vi "Visualise STL file and Octree.vi"() -> ()   [LabVIEW 2017]
doc: "Interactive tool to inspect an STL file and build the Octree for the STL file and check the resulting output. The Octree resolution may be interactively adjusted or set to automatic. The number of branch levels and nodes depends on the geometry, however a rough guide would be to aim for between 5 and 7 branch levels and order 10k nodes."
uses:
  <vilib>/Utility/miscctls.llb/LV3DPointTypeDef.ctl
  <vilib>/Utility/miscctls.llb/LVRGBAColorTypeDef.ctl
  Typedefs/TreeNodeBox.ctl
  Typedefs/Quad.ctl
  Typedefs/Quadplane enum.ctl
  Subroutines/Dot product.vi
panel:
  out "error out":errorcluster
  in  "Camera Controller:Type":T1(ring)=enum."Oriented"
  in  "Autocalc Octree resolution":bool=TRUE
  out "Branch levels":i32
  in  "Scale to unit sphere (render only)":bool
  in  "Octree file path":path=path "C:/EnFlo Software/Anemometry/Anemometry Sub Vis/Collision_Detection/Triangles/Example files/DIPLOS array.oct"
  in  "Render mode":u16(ring)=3 items=["Inherit Value", "Points", "Wireframe", "Polygons"]
  in  "Build Octree":bool
  in  "Draw populated leaf nodes only":bool=TRUE
  out "Number of triangles":u32
  in  "STL file path":path=path "C:/EnFlo Software/Anemometry/Anemometry Sub Vis/Collision_Detection/Triangles/Example files/DIPLOS array.stl"
  in  "Render window":bool=TRUE
  out "Number of Octree nodes":i32
  in  "Octree resolution (model units)":sgl=100.0
  out "Pmin (x, y, z)":sgl[](array[numeric])
  out "Pmax (x, y, z)":sgl[](array[numeric])
  in  "Up Direction":T2={"X"=0.0, "Y"=0.0, "Z"=1.0}
  in  "Target":T2
  in  "Camera Position":T2={"X"=3000.0, "Y"=0.0, "Z"=1000.0}
  out "3D Picture":refnum<vi>(3d-picture)
  # "To view model alone, uncheck \"Build Octree\" and empty \"Octree binary path\".\nTo load Octree after build, uncheck \"Build Octree\"."
  # "PN 03/02/2015"
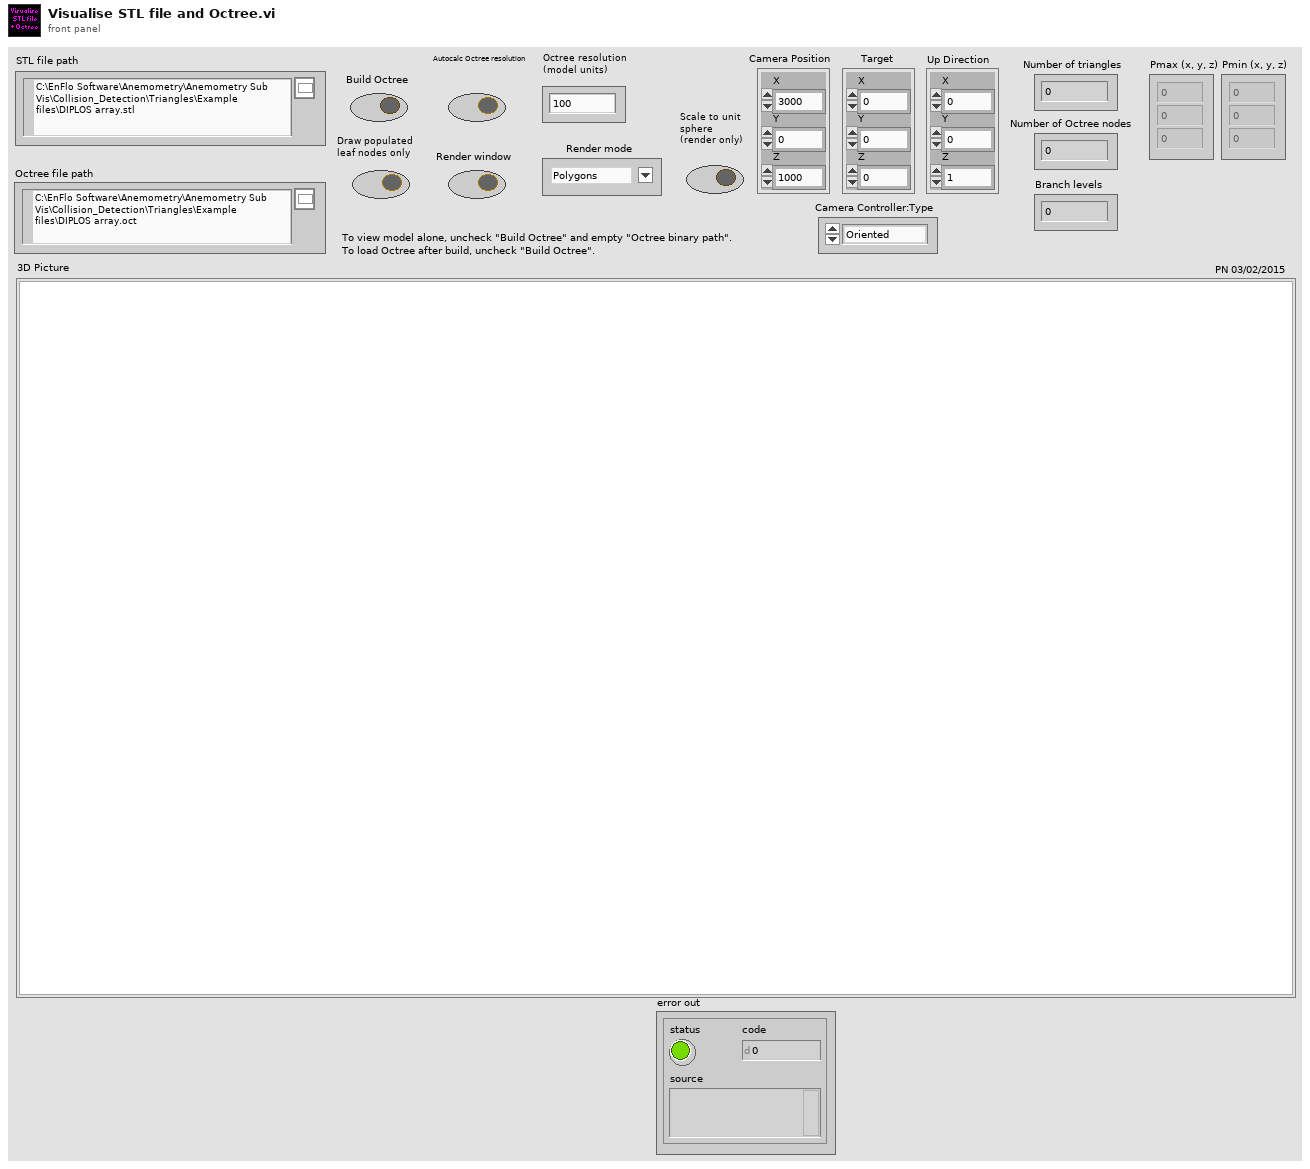
[diagram p1: front panel]
types:
  T1 = enum16{"None", "Spherical", "Flying", "Oriented"}
  T2 = typedef "LV3DPointTypeDef.ctl" = cluster{"X":sgl, "Y":sgl, "Z":sgl}
  T3 = typedef "LVRGBAColorTypeDef.ctl" = cluster{"Red":sgl, "Green":sgl, "Blue":sgl, "Alpha":sgl}
  T4 = typedef "Triangle.ctl" = cluster{"V0":sgl[], "V1":sgl[], "V2":sgl[], "E0":sgl[], "E1":sgl[], "E2":sgl[], "n^":sgl[], "nE0^":sgl[], "nE1^":sgl[], "nE2^":sgl[]}
  T5 = typedef "TreeNodeBox.ctl" = cluster{"Face 0":T6, "Face 1":T6, "Face 2":T6, "Face 3":T6, "Face 4":T6, "Face 5":T6, "Level":i32, "Pmax":sgl[], "Pmin":sgl[], "Parent":i32, "Child 1":i32, "Child 2":i32, "Child 3":i32, "Child 4":i32, "Child 5":i32, "Child 6":i32, "Child 7":i32, "Child 8":i32, "Triangles":i32[], "is leaf node":bool}
  T6 = typedef "Quad.ctl" = cluster{"V0":sgl[], "V1":sgl[], "V2":sgl[], "V3":sgl[], "E0":sgl[], "E1":sgl[], "E2":sgl[], "E3":sgl[], "n^":sgl[], "Plane":T7}
  T7 = typedef "Quadplane enum.ctl" = enum8{"XY", "XZ", "YZ", "-XY", "-XZ", "-YZ"}
  T8 = typedef "LVRectTypeDef.ctl" = cluster{"Left":i16, "Top":i16, "Right":i16, "Bottom":i16}
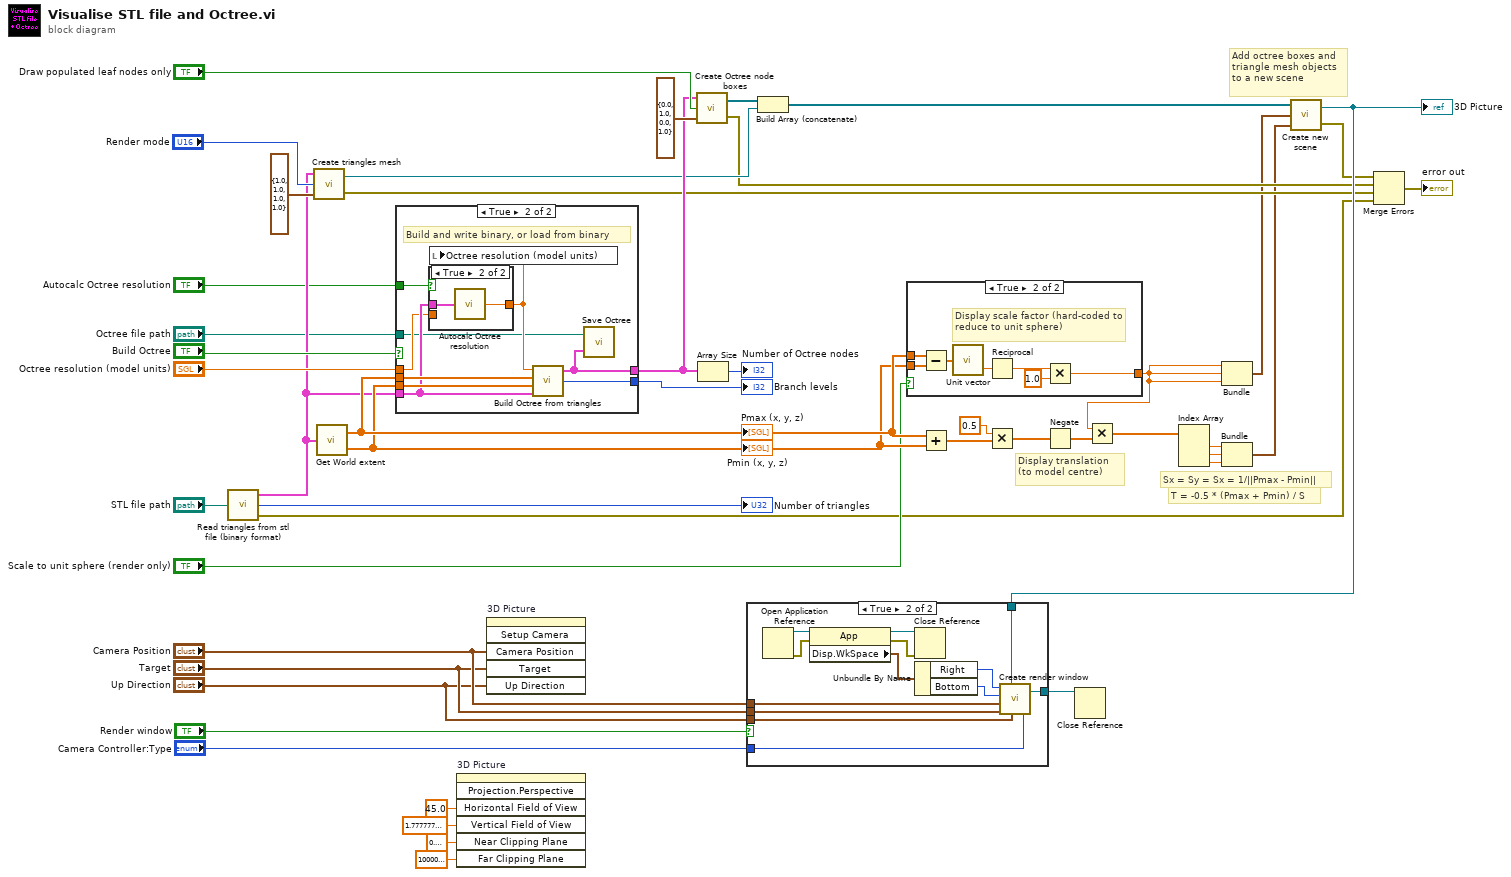
[diagram p0: block diagram]
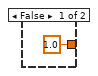
[diagram p3: hidden frame]
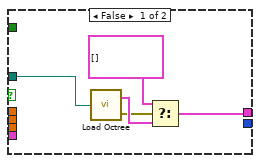
[diagram p4: hidden frame]
diagram:
  # "Add octree boxes and triangle mesh objects to a new scene"
  # "Display translation (to model centre)"
  # "T = -0.5 * (Pmax + Pmin) / S"
  # "Sx = Sy = Sx = 1/||Pmax - Pmin||"
  n1 = call "Read triangles from stl file (binary format).vi"("STL file path"="STL file path") -> ("Triangles array"=w27:T4[], "N triangles"=→"Number of triangles":u32, "Error out"=w5:errorcluster)
  n2 = call "Create triangles mesh.vi"("Colour"=T3 {"Red"=1.0, "Green"=1.0, "Blue"=1.0, "Alpha"=1.0} ("Color"), "Render mode"="Render mode", "Triangles array"=w27) -> ("Error out"=w6:errorcluster, "Triangle mesh out"=w11:refnum<vi>)
  n3 = call "Get World extent.vi"("Triangles"=w27) -> ("Pmax (x, y, z)"=w40:sgl[], "Pmin (x, y, z)"=w39:sgl[])
  "Pmax (x, y, z)" <- w40
  "Pmin (x, y, z)" <- w39
  n4 = case shown="True" "Build Octree" {
    tunnel: "Octree resolution (model units)" -> [_ w55]
    tunnel: w40 -> [_ w61]
    tunnel: w39 -> [_ w60]
    tunnel: [w52 w53] -> w26
    tunnel: w27 -> [_ w57]
    tunnel: "Octree file path" -> [w50 w54]
    tunnel: [_ w59] -> w19
    tunnel: "Autocalc Octree resolution" -> [_ w58]
    frame False {
      n5 = call "Load Octree.vi"("Octree file path"=w50) -> ("Octree node array"=w49:T5[], "Error out"=w48:errorcluster)
      n6 = Select(t=T5[] [], s=w48, f=w49) -> (s? t:f=w52:T5[])
    }
    frame True {
      # "Build and write binary, or load from binary"
      n7 = case shown="True" w58 {
        tunnel: w57 -> [_ w64]
        tunnel: [w62 w63] -> w56
        tunnel: w55 -> [w62 _]
        frame False {
        }
        frame True {
          n8 = call "Autocalc Octree resolution.vi"("Triangles array"=w64) -> ("Suggested resolution"=w63:sgl)
        }
      }
      n9 = local write "Octree resolution (model units)"(w56) -> ()
      n10 = call "Build Octree from triangles.vi"("Triangle array"=w57, "World Pmin (x, y, z)"=w60, "World Pmax (x, y, z)"=w61, "Octree resolution (model units)"=w56) -> ("Branch levels"=w59:i32, "Octree node array"=w53:T5[])  [unwired: 1 out]
      n11 = call "Save Octree.vi"("Octree node array"=w53, "Octree file path"=w54) -> ()  [unwired: 1 out]
    }
  }
  "Branch levels" <- w19
  n12 = invoke on="3D Picture" class="SceneGraphDisp (strict)" method="Projection.Perspective"("Horizontal Field of View"=sgl 45.0 ("Field of View"), "Vertical Field of View"=sgl 1.7777778 ("Aspect Ratio"), "Near Clipping Plane"=sgl 0.1, "Far Clipping Plane"=sgl 1000000.0) -> ()  [unwired: 3 in, 7 out]
  n13 = invoke on="3D Picture" class="SceneGraphDisp (strict)" method="Setup Camera"("Camera Position"="Camera Position", "Target"="Target", "Up Direction"="Up Direction") -> ()  [unwired: 3 in, 6 out]
  n14 = call "Create Octree node boxes.vi"("Colour (emission)"=T3 {"Red"=0.0, "Green"=1.0, "Blue"=0.0, "Alpha"=1.0}, "Draw populated leaf nodes only"="Draw populated leaf nodes only", "Octree nodes array"=w26) -> ("Error out"=w7:errorcluster, "Octree node boxes array"=w12:refnum<vi>[])
  n15 = Array Size(array=w26) -> (size(s)=→"Number of Octree nodes":i32)
  n16 = Build Array (concatenate)(w12, w11) -> (w10:refnum<vi>[])
  n17 = case shown="True" "Scale to unit sphere (render only)" {
    tunnel: w40 -> [_ w72]
    tunnel: w39 -> [_ w71]
    tunnel: [sgl 1.0 w68] -> w36
    frame False {
    }
    frame True {
      # "Display scale factor (hard-coded to reduce to unit sphere)"
      n18 = Subtract(x=w72, y=w71) -> (x-y=w70:sgl[])
      n19 = call "Unit vector.vi"("Vector"=w70) -> ("Vector magnitude"=w67:sgl)  [unwired: 1 out]
      n20 = Reciprocal(x=w67) -> (1/x=w69:sgl)
      n21 = Multiply(x=w69, y=sgl 1.0) -> (x*y=w68:sgl)
    }
  }
  n22 = Add(x=w40, y=w39) -> (x+y=w41:sgl[])
  n23 = Multiply(x=sgl 0.5 ("Numeric"), y=w41) -> (x*y=w35:sgl[])
  n24 = Negate(x=w35) -> (-x=w38:sgl[])
  n25 = Multiply(x=w36, y=w38) -> (x*y=w37:sgl[])
  n26 = Index Array(array=w37) -> (element #1=w45:sgl, element #2=w44:sgl, element #3=w43:sgl)  [unwired: 3 in]
  n27 = Bundle(w36, w36, w36) -> (w3:cluster{sgl, sgl, sgl})  [unwired: 1 in]
  n28 = Bundle(w45, w44, w43) -> (w2:cluster{sgl, sgl, sgl})  [unwired: 1 in]
  n29 = call "Create new scene.vi"("Translation"=w2, "Scale"=w3, "Scene objects array"=w10) -> ("Error out"=w8:errorcluster, "Scene out"=w9:refnum<vi>)
  "3D Picture" <- w9
  n30 = case shown="True" "Render window" {
    tunnel: "Camera Position" -> [_ w86]
    tunnel: "Target" -> [_ w85]
    tunnel: "Up Direction" -> [_ w84]
    tunnel: w9 -> [w73 w83]
    tunnel: "Camera Controller:Type" -> [_ w75]
    tunnel: [w73 w74] -> w1
    frame False {
    }
    frame True {
      n31 = Open Application Reference() -> (0:w79:errorcluster, 3:w78:refnum<vi>)  [unwired: 4 in]
      n32 = property class="App"(reference=w78, error in=w79) -> (reference out=w80:refnum<vi>, error out=w81:errorcluster, "Disp.WkSpace"=w82:T8)
      n33 = Close Reference(reference=w80, error in (no error)=w81) -> ()  [unwired: 1 out]
      n34 = Unbundle By Name(w82) -> ("Right"=w76:i16, "Bottom"=w77:i16)
      n35 = call "Create render window.vi"("Camera Controller:Type"=w75, "Up Direction"=w84, "Scene in"=w83, "Target"=w85, "Camera Position"=w86, "Height"=w77, "Width"=w76) -> ("Scene out"=w74:refnum<vi>)
    }
  }
  n36 = Close Reference(reference=w1) -> ()  [unwired: 1 in, 1 out]
  n37 = Merge Errors(w8, w7, w6, w5) -> (→"error out":errorcluster)
